vi "Functional Global - Temperature Thresholds.vi"(7 "Functional Global Operation (Read)":T1=enum."Read", 11 "Temperature Thresholds in":dbl[](array[numeric])) -> (3 "Temperature Thresholds out":dbl[](array[numeric]))   [LabVIEW 2018]
uses:
  controls/Functional Global Operation.ctl
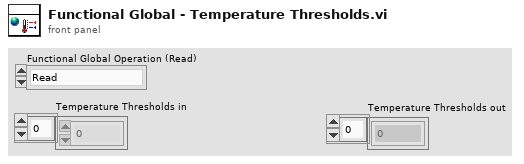
[diagram p1: front panel]
types:
  T1 = typedef "Functional Global Operation.ctl" = enum16{"Initialize", "Read", "Write"}
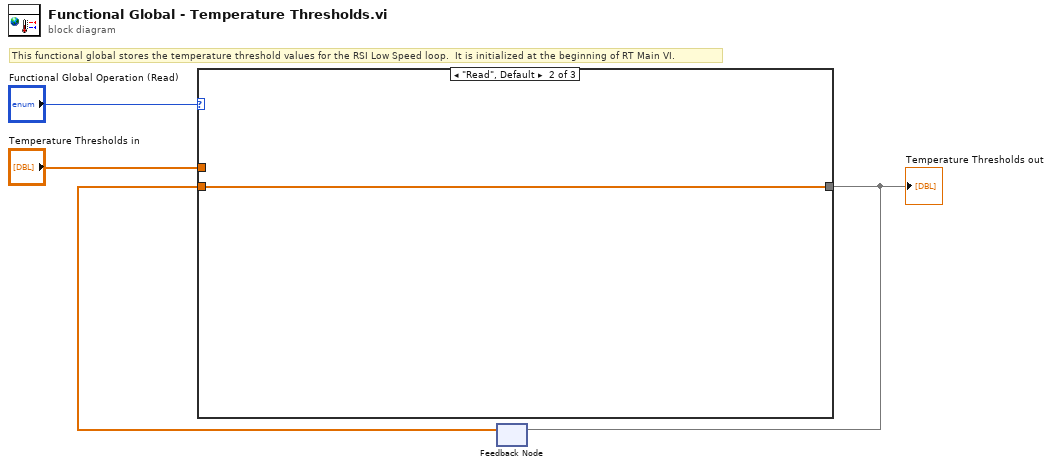
[diagram p0: block diagram]
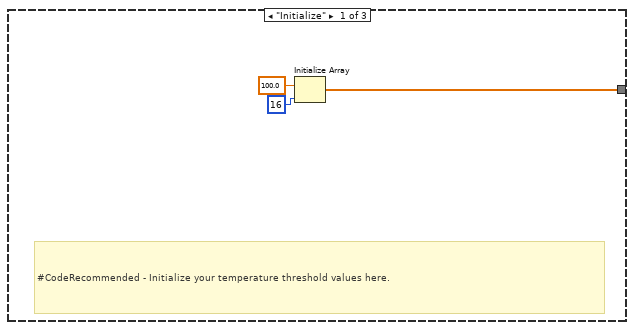
[diagram p2: hidden frame]
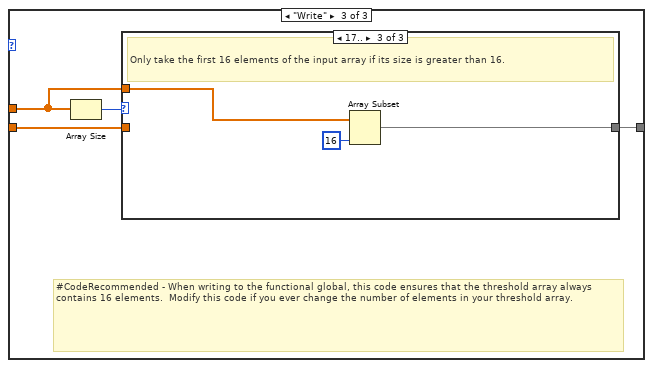
[diagram p3: hidden frame]
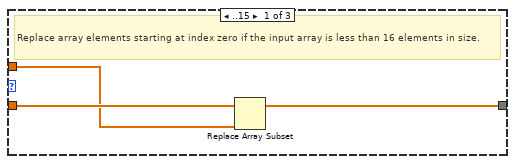
[diagram p4: hidden frame]
diagram:
  # "This functional global stores the temperature threshold values for the RSI Low Speed loop.  It is initialized at the beginning of RT Main VI."
  n1 = feedback #1() -> (w2:dbl[])  [unwired: 1 in]
  n2 = case shown="\"Read\", Default" "Functional Global Operation (Read)" {
    tunnel: "Temperature Thresholds in" -> [_ _ w10]
    tunnel: [w5 w8 w9] -> w1
    tunnel: w2 -> [_ w8 w11]
    frame "Initialize" {
      # "#CodeRecommended - Initialize your temperature threshold values here."
      n3 = Initialize Array(100.0 ("element"), 16 ("dimension size")) -> (w5:dbl[])
    }
    frame "Read", Default {
    }
    frame "Write" {
      # "#CodeRecommended - When writing to the functional global, this code ensures that the threshold array always contains 16 elements.  Modify this code if you ever change the number of elements in your threshold array."
      n4 = Array Size(array=w10) -> (size(s)=w12:i32)
      n5 = case shown="17.." w12 {
        tunnel: w11 -> [w15 _ _]
        tunnel: w10 -> [w14 w16 w19]
        tunnel: [w13 w16 w17] -> w9
        frame ..15 {
          # "Replace array elements starting at index zero if the input array is less than 16 elements in size."
          n6 = Replace Array Subset(array=w15, new element=w14) -> (w13:dbl[])  [unwired: 1 in]
        }
        frame 16, Default {
          # "The input array has exactly 16 elements."
        }
        frame 17.. {
          # "Only take the first 16 elements of the input array if its size is greater than 16."
          n7 = Array Subset(array=w19, length=16) -> (w17:dbl[])  [unwired: 1 in]
        }
      }
    }
  }
  "Temperature Thresholds out" <- w1
  n8 = feedback-in #1(w1) -> ()
